vi "Frame_to_word_Felica.vi"() -> ()   [LabVIEW 2019]
uses:
  <vilib>/addons/Modulation/Analog/support/mod_Set Error Source.vi
  <vilib>/addons/Modulation/Digital/Support/Common/Validators/mod_Generate Filter Coefficients Validate.vi
  <vilib>/addons/Modulation/Digital/General/subVIs/mod_Generate Filter Coefficients.vi
  <vilib>/addons/Modulation/Digital/General/MT Generate ASK system parameters (M).vi
  <vilib>/addons/Modulation/Analog/MT Modulate AM (DSB).vi
  <vilib>/addons/Modulation/Analog/MT Upconvert Baseband (Real).vi
  <vilib>/measure/macond.llb/IIR Filter for 1 Chan.vi
  <vilib>/express/express analysis/Spectral/Block/exnSpectralBlock spectral measurements RMS poly.vi
  <vilib>/express/express analysis/Spectral/Block/exnSpectralBlock spectral measurements RMS WFM.vi
  <vilib>/addons/Modulation/Analog/MT Downconvert Passband (Real).vi
  <vilib>/addons/Modulation/Analog/MT Demodulate AM (DSB).vi
  <vilib>/ErrorRing/Error Ring.xnode
  <vilib>/express/express analysis/Spectral/XNode/ExpressSpectralMeasurementsBlockNode.xnode
  <vilib>/addons/Modulation/niAMT.lvlib
  <vilib>/measure/NI_MAPro.lvlib
  <vilib>/addons/Modulation/niDMT.lvlib
panel:
  out "DEMODulate 2":cluster{"t0":dbl, "dt":dbl, "Y":dbl[]}(graph)
  out "Array of byte":u8[](array[numeric]) format="%x"
  out "decode":cluster{"t0":dbl, "dt":dbl, "Y":dbl[]}(graph)
  out "Command":cluster{"t0":dbl, "dt":dbl, "Y":dbl[]}(graph)
  out "DEMODulate":cluster{"t0":dbl, "dt":dbl, "Y":dbl[]}(graph)
  out "spectrum analog signal 6":waveform(dbl)(graph)
  out "spectrum analog signal 5":cluster{"t0":dbl, "dt":dbl, "Y":dbl[]}(graph)
  out "Analog signal 8":waveform(dbl)(graph)
  out "spectrum analog signal 4":cluster{"t0":dbl, "dt":dbl, "Y":dbl[]}(graph)
  out "antenna":waveform(dbl)(graph)
  out "summ":waveform(dbl)(graph)
  out "antenna 2":waveform(dbl)(graph)
  out "spectrum analog signal 3":cluster{"t0":dbl, "dt":dbl, "Y":dbl[]}(graph)
  out "spectrum analog signal 2":cluster{"t0":dbl, "dt":dbl, "Y":dbl[]}(graph)
  out "spectrum analog signal":cluster{"t0":dbl, "dt":dbl, "Y":dbl[]}(graph)
  in  "nfcid":u8[](array[numeric])=[1, 2, 3, 4, 5, 1, 2, 3, 4, 5] format="%x"
  in  "DID":u8[](array[numeric])=[20] format="%x"
  in  "CMD2":u8[](array[numeric])=[2] format="%x"
  in  "CMD1":u8[](array[numeric])=[212] format="%x"
  out "Video  without CRC":cluster{"t0":dbl, "dt":dbl, "Y":dbl[]}(graph)
  out "CRC out":u16 format="%x"
  in  "Preambul":u8[](array[numeric])=[0, 0, 0, 0, 0, 0] format="%x"
  in  "SYNC":u8[](array[numeric])=[178, 212] format="%x"
  out "Video":cluster{"t0":dbl, "dt":dbl, "Y":dbl[]}(graph)
  out "video Manchecter":cluster{"t0":dbl, "dt":dbl, "Y":dbl[]}(graph)
  in  "command":enum16{"WUP_REQ", "REQB"}(ring)
  in  "CARRIER (hz)":dbl
  in  "BIT RATE":dbl
  out "10% ASK":waveform(dbl)(graph)
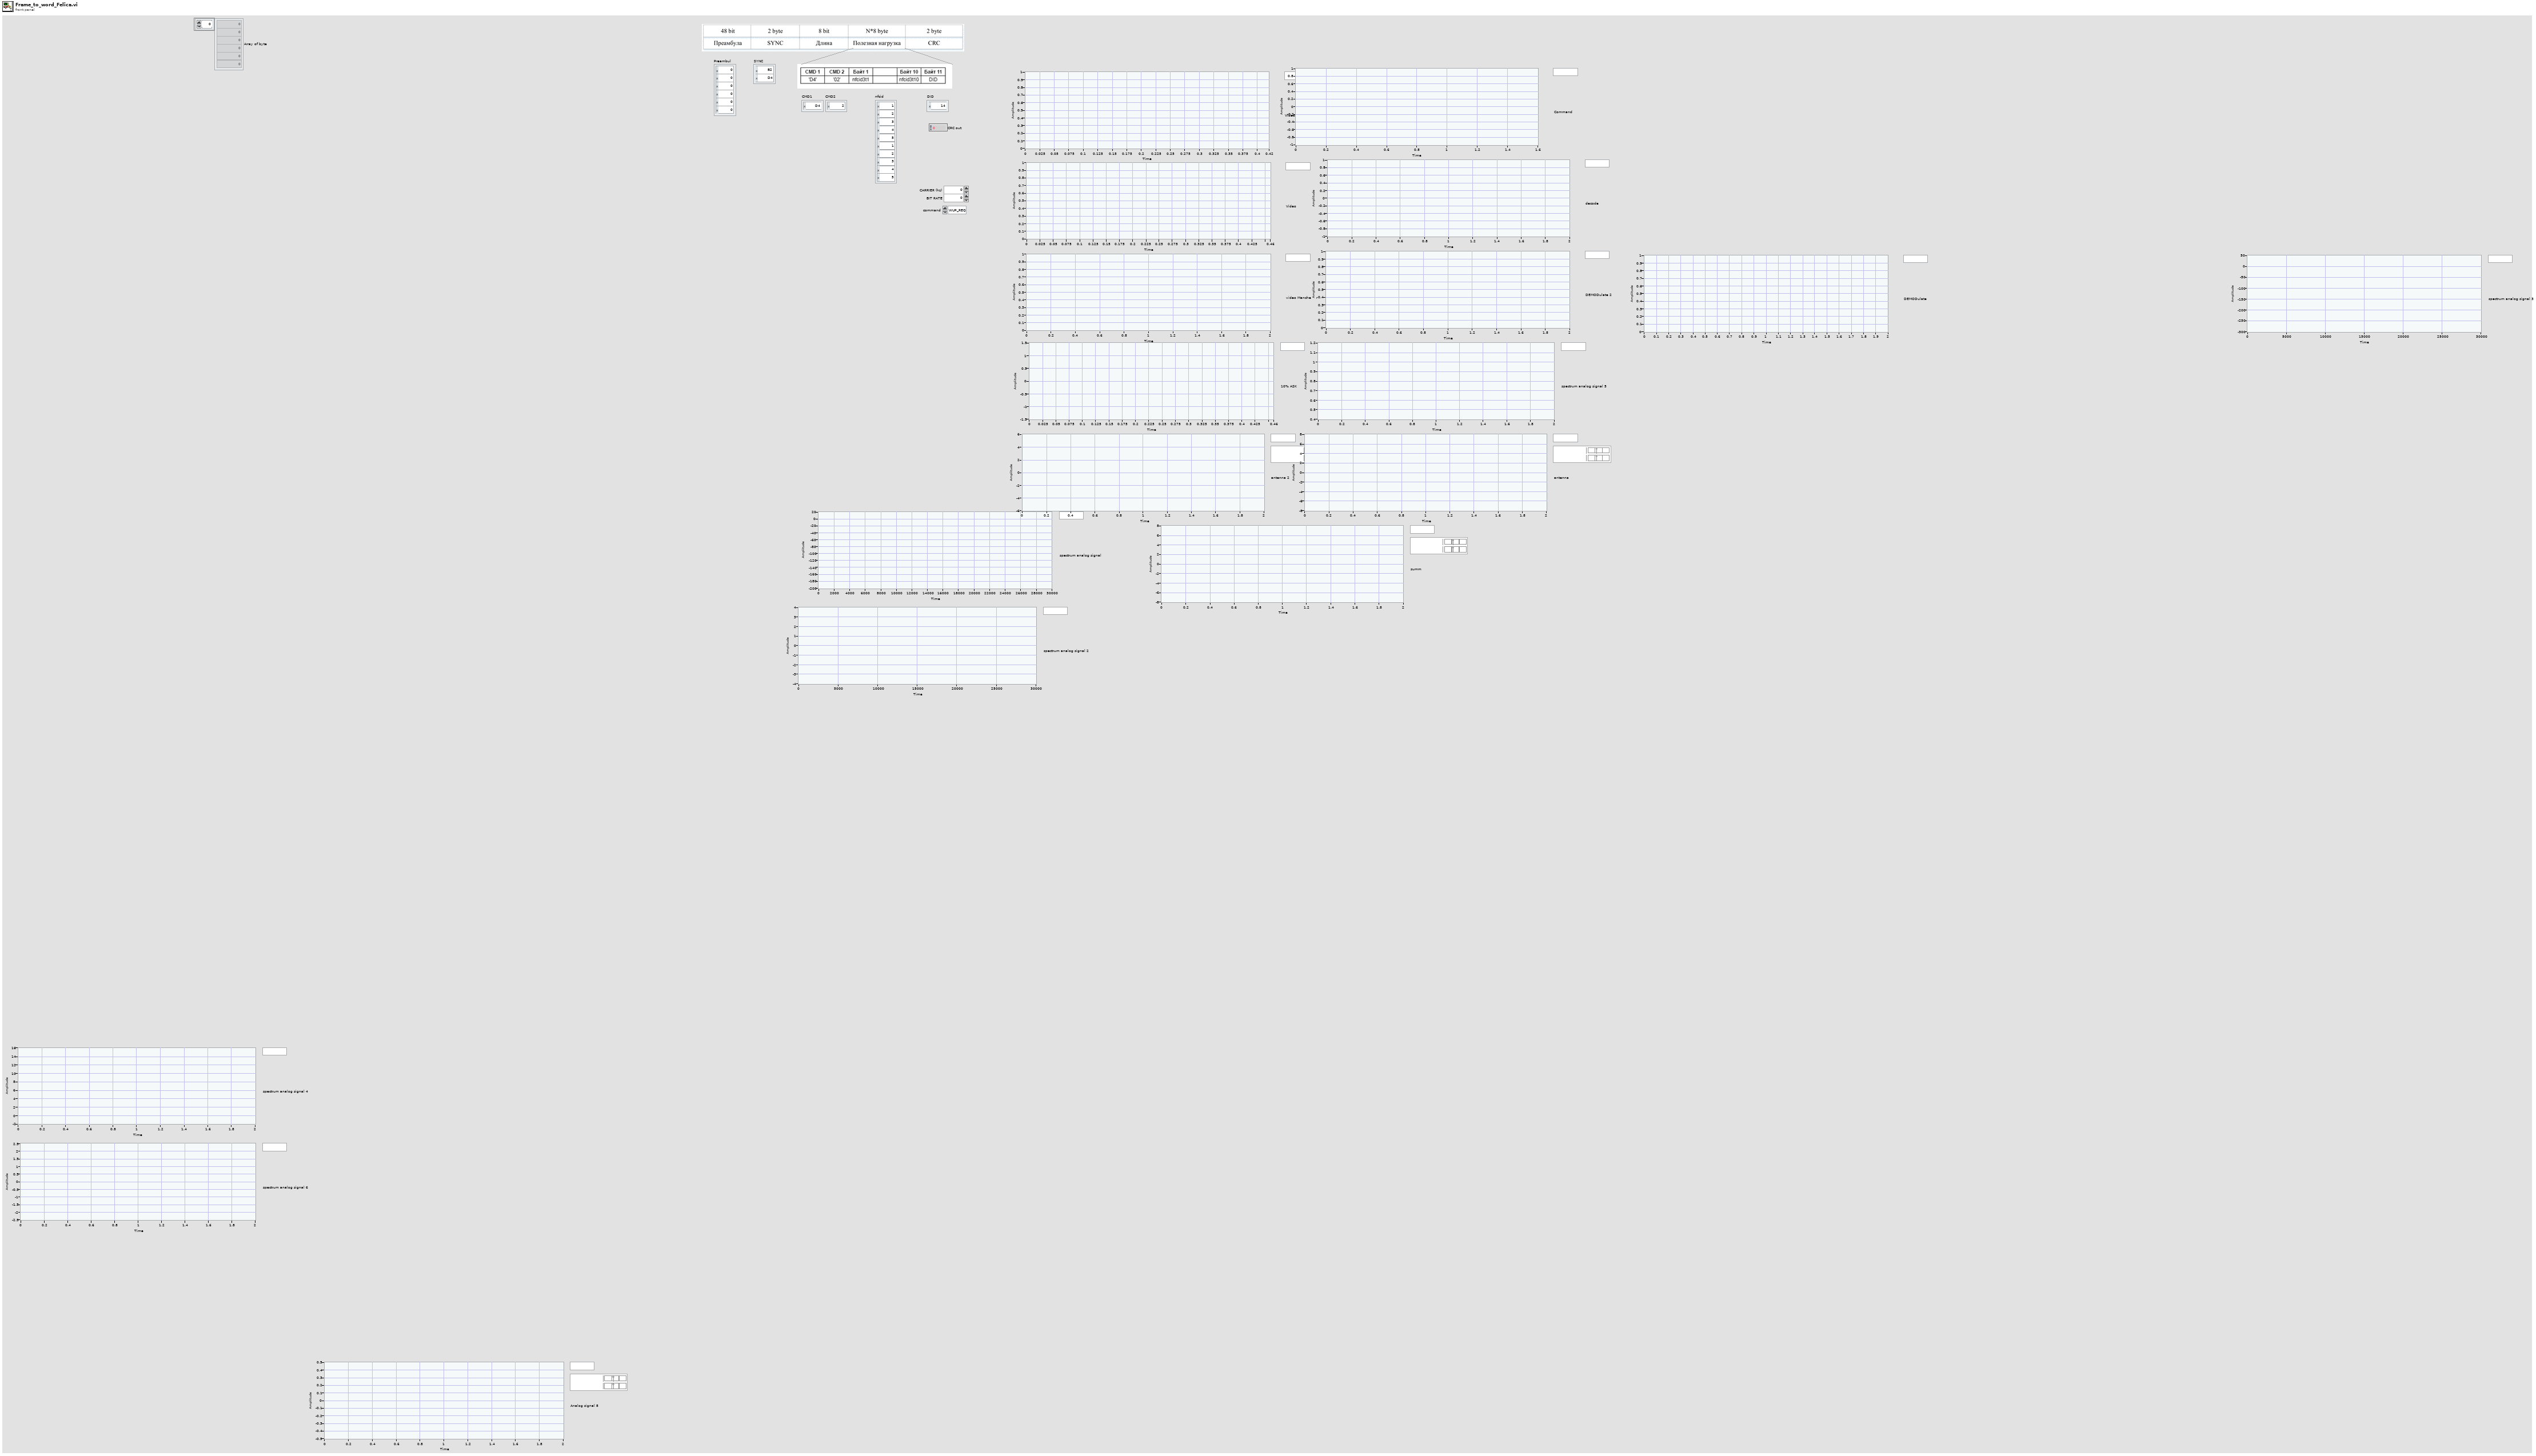
[diagram p1: front panel]
types:
  T1 = enum16{"none", "Raised Cosine", "Root Raised Cos", "Gaussian"}
  T2 = enum16{"FSK", "PSK", "QAM", "MSK", "PAM", "ASK", "CPM"}
  T3 = cluster{"Topology":enum16{"Off", "Butterworth", "Chebyshev", "Inverse Chebyshev", "Elliptic", "Bessel"}, "Type":enum16{"Lowpass", "Highpass", "Bandpass", "Bandstop"}, "Order":i32, "Lower Fc":dbl, "Upper Fc":dbl, "PB Ripple":dbl, "SB Attenuation":dbl}
  T4 = cluster{"passband ripple (dB)":dbl, "stopband start (Hz)":dbl, "stopband gain (dB)":dbl, "compute filter stopband ? (T)":bool}
  T5 = typedef "niAMT.lvlib/Complex Data Waveform.ctl" = cluster{"t0":dbl, "dt":dbl, "Y":cdb[]}
  T6 = cluster{"samples per symbol (16)":i32, "symbol map":cdb[]}
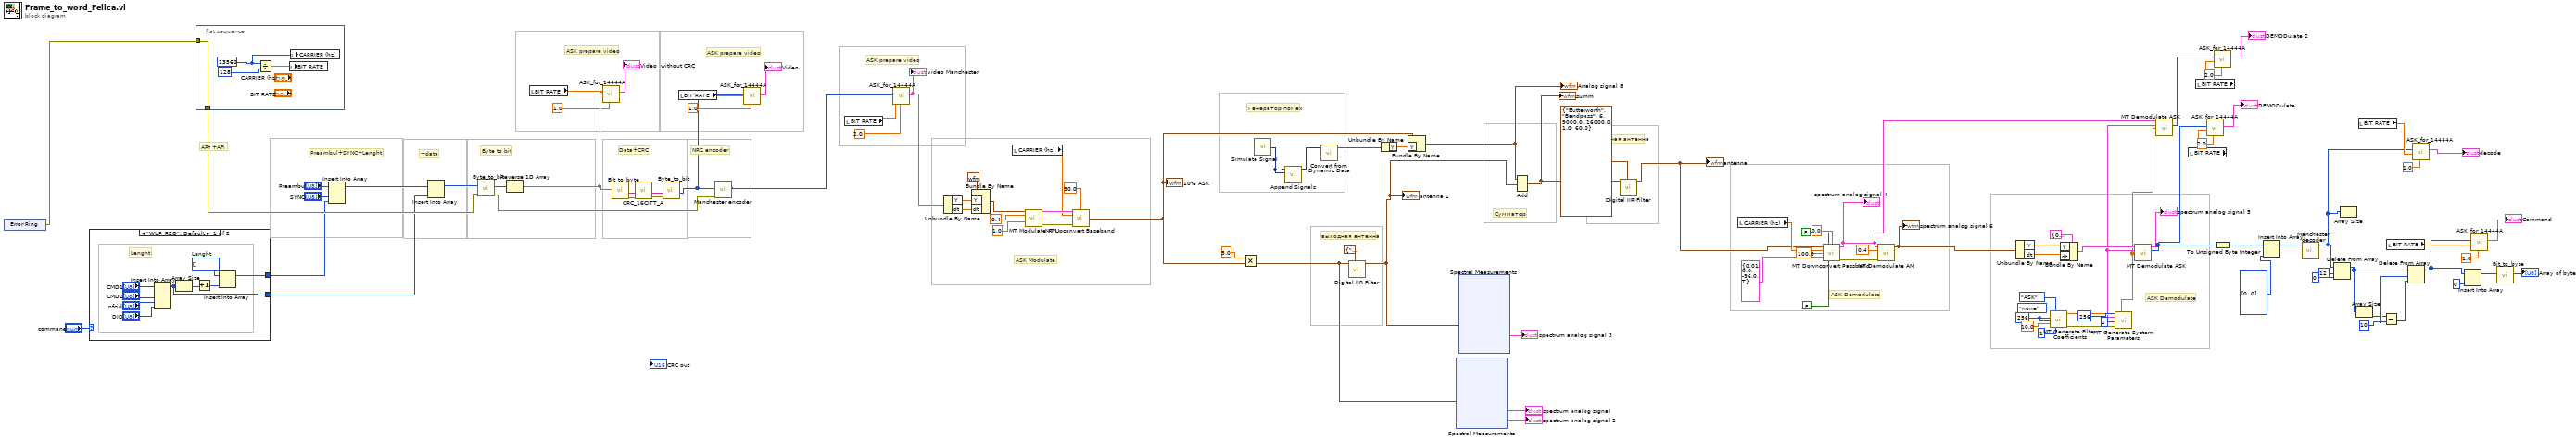
[diagram p0: block diagram]
diagram:
  w25 = 10 ("length")
  w53 = 256 ("pulse shaping samples per symbol (16)")
  # "ASK Demodulate"
  # "ASK Demodulate"
  # "входная антенна"
  # "Сумматор"
  # "выходная антенна"
  # "Генератор помех"
  # "+data"
  # "Preambul+SYNC+Lenght"
  # "ASK prepare video"
  # "Data+CRC"
  # "APf +AFi"
  # "ASK Modulate"
  # "ASK prepare video"
  # "ASK prepare video"
  # "NRZ encoder"
  # "Byte to bit"
  n1 = xnode "Error Ring"() -> ("error out"=w90:errorcluster)
  n2 = case shown="\"WUP_REQ\", Default" "command" {
    tunnel: [w108 _] -> w81
    tunnel: [w107 _] -> w78
    frame "WUP_REQ", Default {
      w110 = u8[] []  # Lenght
      # "Lenght"
      n3 = Insert Into Array(array="CMD1", new element #1="CMD2", new element #2="nfcid", new element #3="DID") -> (w107:u8[])  [unwired: 1 in]
      n4 = Array Size(array=w107) -> (size(s)=w111:i32)
      n5 = Increment(x=w111) -> (x+1=w109:i32)
      n6 = Insert Into Array(array=w110, new element=w109) -> (w108:u8[])  [unwired: 1 in]
    }
    frame "REQB" {
    }
  }
  n7 = flat-sequence {
    tunnel: w90 -> [w116]
    tunnel: [w116] -> w89
    frame #0 {
      w117 = u32 13560
      n8 = Divide(x=w117, y=u32 128) -> (x/y=w118:dbl)
      n9 = local write "BIT RATE"(w118) -> ()
      n10 = local write "CARRIER (hz)"(w117) -> ()
    }
  }
  n11 = Insert Into Array(array="Preambul", new element #1="SYNC", new element #2=w81) -> (w80:u8[])  [unwired: 1 in]
  n12 = Insert Into Array(array=w80, new element=w78) -> (w79:u8[])  [unwired: 1 in]
  n13 = call "Byte_to_bit.vi"("Error In"=w89, "Array of byte"=w79) -> ("Error Out"=w75:errorcluster, "Arrray of bit"=w106:u8[])  [unwired: 5 in, 1 out]
  n14 = Reverse 1D Array(array=w106) -> (reversed array=w103:u8[])
  n15 = local read "BIT RATE"() -> (w84:dbl)
  n16 = call "ASK_for_14444A.vi"("encoder divider"=1.0 ("y"), "BIT RATE"=w84, "Bit stream out (NRZ encode)"=w103) -> ("output complex waveform"=→"Video  without CRC":T5)  [unwired: 7 in, 1 out]
  n17 = call "Bit_to_byte.vi"("Array of bit"=w103) -> ("Error Out"=w72:errorcluster, "BYTE"=w71:string)  [unwired: 8 in, 1 out]
  n18 = call "CRC_16CITT_A.vi"("Error In"=w72, "DATA PACKET"=w71) -> ("Error Out"=w77:errorcluster, "DATA PACKET+CRC"=w70:string)  [unwired: 5 in, 1 out]
  n19 = call "Byte_to_bit.vi"("Error In"=w77, "BYTE"=w70) -> ("Arrray of bit (str)"=w76:u8[])  [unwired: 5 in, 2 out]
  n20 = local read "BIT RATE"() -> (w96:dbl)
  n21 = call "Manchester encoder.vi"("Error In"=w75, "Bit stream in"=w76) -> ("Bit stream out (Manchester encode)"=w74:u8[])  [unwired: 8 in, 1 out]
  n22 = call "ASK_for_14444A.vi"("encoder divider"=1.0 ("y"), "BIT RATE"=w96, "Bit stream out (NRZ encode)"=w76) -> ("output complex waveform"=→"Video":T5)  [unwired: 7 in, 1 out]
  n23 = local read "BIT RATE"() -> (w105:dbl)
  n24 = call "ASK_for_14444A.vi"("encoder divider"=2.0 ("y"), "BIT RATE"=w105, "Bit stream out (NRZ encode)"=w74) -> ("output complex waveform"=w73:T5)  [unwired: 7 in, 1 out]
  "video Manchecter" <- w73
  n25 = Unbundle By Name(w73) -> ("Y"=w93:cdb[], "dt"=w92:dbl)
  n26 = Bundle By Name(cluster=waveform(cdb) {"t0"=timestamp(0 s since 1904-01-01), "dt"=1.0, "Y"=[]} ("waveform"), "Y"=w93, "dt"=w92) -> (w99:waveform(cdb))
  n27 = local read "CARRIER (hz)"() -> (w97:dbl)
  n28 = call-poly <vilib>:"MT Modulate AM.vi"("message signal"=w99, "modulation index"=0.4, "peak message amplitude"=1.0) -> ("AM modulated waveform"=w98:cluster{"t0":dbl, "dt":dbl, "Y":cdb[]}, "error out"=w101:errorcluster)  [unwired: 11 in]
  n29 = call-poly <vilib>:"MT Upconvert Baseband.vi"("baseband waveform (complex)"=w98, "initial phase (deg)"=90.0, "carrier frequency (Hz)"=w97, "error in (no error)"=w101) -> ("passband waveform"=w12:waveform(dbl))  [unwired: 10 in, 1 out]
  "10% ASK" <- w12
  n30 = Multiply(x=5.0, y=w12) -> (x*y=w14:waveform(dbl))
  n31 = call "Simulate Signal"() -> ("Sine with Gaussian Noise"=w4:dynamicdata)  [unwired: 14 in, 1 out]
  n32 = call "Append Signals"("Input Signal B"=w4, "Input Signal A"=w4) -> ("Appended Signals"=w3:dynamicdata)  [unwired: 8 in, 1 out]
  n33 = call "Convert from Dynamic Data"("Dynamic Data Type"=w3) -> ("Waveform"=w65:waveform(dbl))  [unwired: 3 in]
  n34 = call-poly <vilib>:"Digital IIR Filter.vi"("IIR filter specifications"=T3 {"Topology"=enum."Butterworth", "Type"=enum."Bandpass", "Order"=3, "Lower Fc"=9000.0, "Upper Fc"=16000.0, "PB Ripple"=1.0, "SB Attenuation"=60.0}, "signal in"=w14) -> ("signal out"=w58:waveform(dbl))  [unwired: 7 in, 2 out]
  "antenna 2" <- w58
  n35 = Unbundle By Name(w65) -> ("Y"=w64:dbl[])
  n36 = Bundle By Name(cluster=w12, "Y"=w64) -> (w57:waveform(dbl))
  "Analog signal 8" <- w57
  n37 = xnode "Spectral Measurements"("Signals"=w14) -> ("FFT - (RMS)"=→"spectrum analog signal":cluster{"f0":dbl, "df":dbl, "magnitude":dbl[]}, "Phase"=→"spectrum analog signal 2":cluster{"f0":dbl, "df":dbl, "phase":dbl[]})  [unwired: 1 in, 1 out]
  n38 = xnode "Spectral Measurements"("Signals"=w58) -> ("FFT - (RMS)"=→"spectrum analog signal 3":cluster{"f0":dbl, "df":dbl, "magnitude":dbl[]})  [unwired: 1 in, 2 out]
  n39 = Add(1:w58, 2:w57) -> (0:w62:waveform(dbl))  [unwired: 1 in, 1 out]
  "summ" <- w62
  n40 = call-poly <vilib>:"Digital IIR Filter.vi"("IIR filter specifications"=T3 {"Topology"=enum."Butterworth", "Type"=enum."Bandpass", "Order"=6, "Lower Fc"=9000.0, "Upper Fc"=16000.0, "PB Ripple"=1.0, "SB Attenuation"=60.0}, "signal in"=w62) -> ("signal out"=w42:waveform(dbl))  [unwired: 7 in, 2 out]
  "antenna" <- w42
  n41 = local read "CARRIER (hz)"() -> (w61:dbl)
  n42 = call-poly <vilib>:"MT Downconvert Passband.vi"("Waveform"=w42, "reset? (F)"=FALSE, "initial phase (deg)"=0.0, "carrier frequency (Hz)"=w61, "passband bandwidth (Hz)"=100.0, "advanced filter parameters"=T4 {"passband ripple (dB)"=0.01, "stopband start (Hz)"=0.0, "stopband gain (dB)"=-96.0, "compute filter stopband ? (T)"=TRUE}, "enable filter (T)"=FALSE) -> ("downconverted waveform (complex baseband)"=w11:T5, "error out"=w43:errorcluster)  [unwired: 5 in, 2 out]
  "spectrum analog signal 4" <- w11
  n43 = call-poly <vilib>:"MT Demodulate AM.vi"("AM modulated waveform"=w11, "modulation index"=0.4, "error in (no error)"=w43) -> ("AM demodulated waveform"=w41:waveform(dbl))  [unwired: 10 in, 2 out]
  "spectrum analog signal 6" <- w41
  n44 = Unbundle By Name(w41) -> ("Y"=w39:dbl[], "dt"=w38:dbl)
  n45 = call <vilib>:"MT Generate Filter Coefficients.vi"("pulse shaping filter (none)"=T1."none", "modulation type"=T2."ASK", "pulse shaping samples per symbol (16)"=w53, "matched samples per symbol (16)"=w53, "filter parameter"=10.0, "filter length (symbols)"=1) -> ("pulse shaping filter coefficients"=w9:dbl[], "error out"=w50:errorcluster)  [unwired: 1 in, 7 out]
  n46 = Bundle By Name(cluster=cluster{"t0":dbl, "dt":dbl, "Y":dbl[]} {"t0"=0.0, "dt"=0.0, "Y"=[]} ("AM modulated waveform"), "Y"=w39, "dt"=w38) -> (w37:cluster{"t0":dbl, "dt":dbl, "Y":dbl[]})
  n47 = call-poly <vilib>:"MT Generate System Parameters.vi"("samples per symbol (16)"=256, "M-ASK (2)"=2, "error in (no error)"=w50) -> ("ASK system parameters"=w10:T6)  [unwired: 12 out]
  n48 = call <vilib>:"MT Demodulate ASK.vi"("input complex waveform"=w37, "ASK system parameters"=w10, "matched filter coefficients"=w9) -> ("recovered complex waveform"=→"spectrum analog signal 5":T5, "output bit stream"=w31:i8[])  [unwired: 8 in, 3 out]
  n49 = call <vilib>:"MT Demodulate ASK.vi"("input complex waveform"=w11, "ASK system parameters"=w10, "matched filter coefficients"=w9) -> ("output bit stream"=w5:i8[])  [unwired: 8 in, 4 out]
  n50 = local read "BIT RATE"() -> (w34:dbl)
  n51 = local read "BIT RATE"() -> (w8:dbl)
  n52 = call "ASK_for_14444A.vi"("encoder divider"=2.0 ("y"), "BIT RATE"=w34, "Bit stream out (NRZ encode)"=w31) -> ("output complex waveform"=→"DEMODulate":T5)  [unwired: 7 in, 1 out]
  n53 = call "ASK_for_14444A.vi"("encoder divider"=2.0 ("y"), "BIT RATE"=w8, "Bit stream out (NRZ encode)"=w5) -> ("output complex waveform"=→"DEMODulate 2":T5)  [unwired: 7 in, 1 out]
  n54 = To Unsigned Byte Integer(number=w31) -> (unsigned 8bit integer=w21:u8[])
  n55 = Insert Into Array(array=w21, new element=u8[] [0, 0]) -> (w2:u8[])  [unwired: 1 in]
  n56 = call "Manchester decoder.vi"("Bit stream in"=w2) -> ("Array"=w1:u8[])  [unwired: 9 in, 1 out]
  n57 = Delete From Array(array=w1, length=12, index=0) -> (array with subset deleted=w27:u8[])  [unwired: 1 out]
  n58 = Array Size(array=w1) -> ()  [unwired: 1 out]
  n59 = Array Size(array=w27) -> (size(s)=w23:i32)
  n60 = local read "BIT RATE"() -> (w33:dbl)
  n61 = Subtract(x=w23, y=w25) -> (x-y=w24:i32)
  n62 = local read "BIT RATE"() -> (w28:dbl)
  n63 = Delete From Array(array=w27, length=w25, index=w24) -> (array with subset deleted=w18:u8[])  [unwired: 1 out]
  n64 = call "ASK_for_14444A.vi"("encoder divider"=1.0 ("y"), "BIT RATE"=w33, "Bit stream out (NRZ encode)"=w1) -> ("output complex waveform"=→"decode":T5)  [unwired: 7 in, 1 out]
  n65 = Insert Into Array(array=w18, new element=u8 0 ("new element/subarray")) -> (w16:u8[])  [unwired: 1 in]
  n66 = call "ASK_for_14444A.vi"("encoder divider"=1.0 ("y"), "BIT RATE"=w28, "Bit stream out (NRZ encode)"=w18) -> ("output complex waveform"=→"Command":T5)  [unwired: 7 in, 1 out]
  n67 = call "Bit_to_byte.vi"("Array of bit"=w16) -> ("Array of byte"=→"Array of byte":u8[])  [unwired: 8 in, 2 out]
